vi "Create Resources.vi"() -> ()   [LabVIEW 2017, in "GPIO.lvlib" / "GPIO.lvclass"]
uses:
  GPIO.lvclass
  <vilib>/rvi/LocalResourceManager/LocalResourceManager.xnode
  <vilib>/rvi/DataTransferAndStorage/Container/Common/niFpgaContainerGetUniqueNameForEmu.vi
  <vilib>/rvi/DataTransferAndStorage/Container/Common/niFpgaContainerSetEmuInfo.vi
  <vilib>/rvi/eio/common/nirviEmuReportErrorAndStop.vi
  <instrlib>/_niInstr/Instruction Framework/v1/FPGA/Interfaces/Address Space/Address Space.lvclass
  <instrlib>/_niInstr/Instruction Framework/v1/FPGA/Helper Classes/Single Address Space Collection/Single Address Space Collection.lvclass
  C:/Program Files (x86)/National Instruments/LabVIEW 2017/instr.lib/_niInstr/Instruction Framework/v1/FPGA/Interfaces/Address Space/Address Space.lvclass
panel:
  out "gpio subsystem":refnum<class "Single Address Space Collection.lvclass">
  out "gpio address space":refnum<class "GPIO.lvclass">
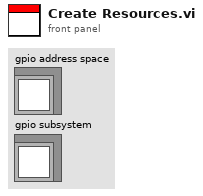
[diagram p1: front panel]
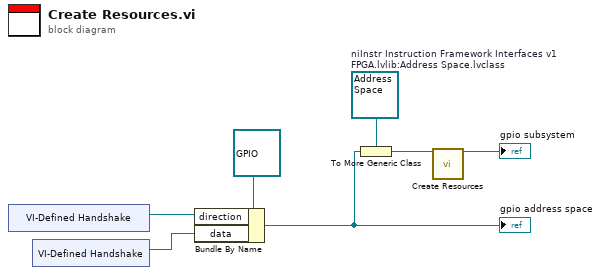
[diagram p0: block diagram]
diagram:
  w3 = refnum<class "Address Space.lvclass"> refnum  # niInstr Instruction Framework Interfaces v1 FPGA.lvlib:Address Space.lvclass
  n1 = xnode "VI-Defined Handshake"() -> ("Handshake Out"=w6:refnum<k21>)
  n2 = xnode "VI-Defined Handshake"() -> ("Handshake Out"=w5:refnum<k21>)
  n3 = Bundle By Name(cluster=refnum<class "GPIO.lvclass"> refnum ("GPIO.lvclass"), "direction"=w6, "data"=w5) -> (w4:refnum<class "GPIO.lvclass">)
  "gpio address space" <- w4
  n4 = To More Generic Class(target class=w3, reference=w4) -> (generic class reference=w2:refnum<class "Address Space.lvclass">)
  n5 = call "Create Resources.vi"("address space"=w2) -> ("single address space collection"=→"gpio subsystem":refnum<class "Single Address Space Collection.lvclass">)  [unwired: 14 in]
